vi "Start Process.vi"(8 "error in":errorcluster, 10 "Execution Plan":T1={"Exe Path"=path "", "Args"=[], "Timeout"=-1}, 11 "Process Executor in":refnum<class "Process Executor.lvclass">) -> (0 "error out":errorcluster, 3 "Process Executor out":refnum<class "Process Executor.lvclass">)   [LabVIEW 2025, in "Process Executor.lvclass"]
doc: "Creates a complete ProcessStartInfo structure from a provided Execution Plan and starts the specified external process accordingly."
uses:
  Process Executor.lvclass
  Type Definitions/Execution Plan--cluster.ctl
  Process Executor.lvclass/Process Executor.ctl
  C:/Program Files (x86)/dotnet/shared/Microsoft.NETCore.App/8.0.23/System.Diagnostics.Process.dll
  Program Files (x86)/dotnet/shared/Microsoft.NETCore.App/8.0.23/System.Diagnostics.Process.dll
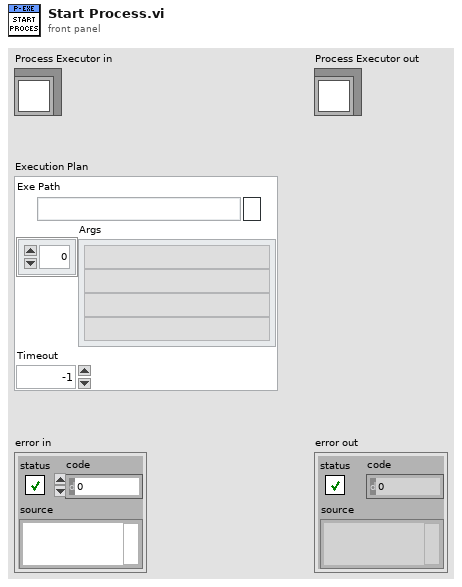
[diagram p1: front panel]
types:
  T1 = typedef "Execution Plan--cluster.ctl" = cluster{"Exe Path":path, "Args":string[], "Timeout":i32}
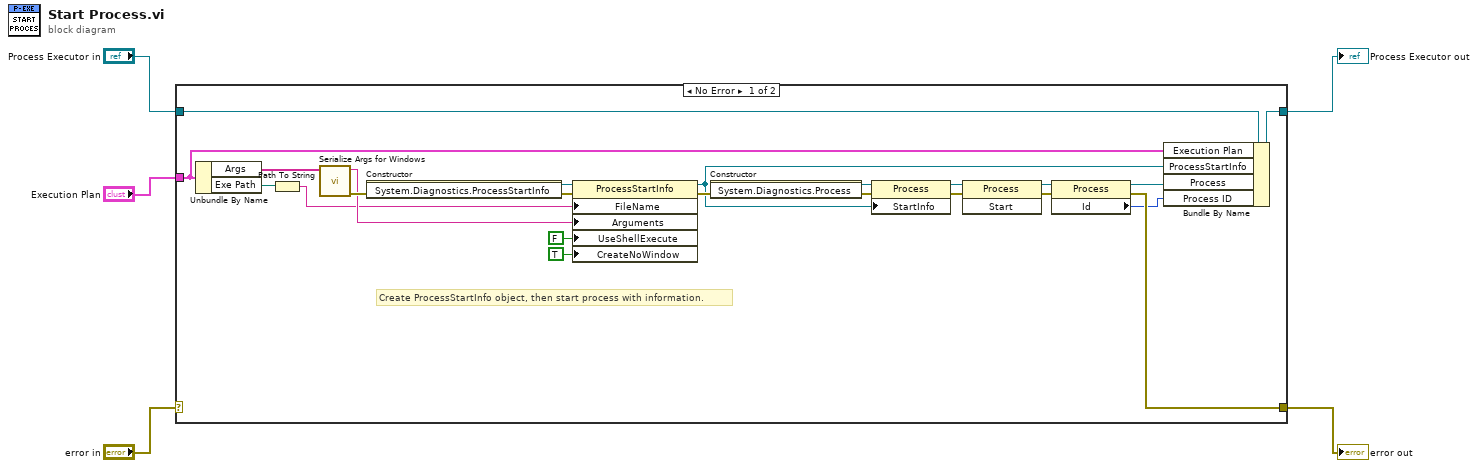
[diagram p0: block diagram]
diagram:
  n1 = case shown="No Error" "error in" {
    selector: "error in" -> [_ w30]
    tunnel: [w22 w30] -> w4
    tunnel: [w12 w29] -> w2
    tunnel: "Process Executor in" -> [w11 w29]
    tunnel: "Execution Plan" -> [w9 _]
    frame No Error {
      # "Create ProcessStartInfo object, then start process with information."
      n2 = Unbundle By Name(w9) -> ("Args"=w21:string[], "Exe Path"=w14:path)
      n3 = Path To String(path=w14) -> (string=w13:string)
      n4 = call "Serialize Args for Windows.vi"("Args"=w21) -> ("error out"=w24:errorcluster, "String"=w15:string)  [unwired: 9 in]
      n5 = constructor class="ProcessStartInfo" ("Constructor Node")(error in=w24) -> (reference out=w18:refnum<k39>, error out=w25:errorcluster)  [unwired: 2 in, 1 out]
      n6 = property on="Property Node" class="ProcessStartInfo"(reference=w18, error in=w25, "FileName"=w13, "Arguments"=w15, "UseShellExecute"=FALSE, "CreateNoWindow"=TRUE) -> (reference out=w10:refnum<k39>, error out=w27:errorcluster)
      n7 = constructor class="Process" ("Constructor Node")(error in=w27) -> (reference out=w19:refnum<k39>, error out=w26:errorcluster)  [unwired: 2 in, 1 out]
      n8 = property on="Property Node" class="Process"(reference=w19, error in=w26, "StartInfo"=w10) -> (reference out=w20:refnum<k39>, error out=w28:errorcluster)
      n9 = invoke on="Invoke Node" class="Process" method="Start"(reference=w20, error in=w28) -> (reference out=w8:refnum<k39>, error out=w23:errorcluster)  [unwired: 1 in, 1 out]
      n10 = property class="Process"(reference=w8, error in=w23) -> (reference out=w7:refnum<k39>, error out=w22:errorcluster, "Id"=w6:i32)
      n11 = Bundle By Name(cluster=w11, "Execution Plan"=w9, "ProcessStartInfo"=w10, "Process"=w7, "Process ID"=w6) -> (w12:refnum<class "Process Executor.lvclass">)
    }
    frame Error {
    }
  }
  "error out" <- w4
  "Process Executor out" <- w2
